vi "Open UI.vi"(11 "Open UI in":refnum<class "Open UI.lvclass">) -> (0 "error out":errorcluster, 3 "Open UI out":refnum<class "Open UI.lvclass">)   [LabVIEW 2021, in "Open UI.lvlib" / "Open UI.lvclass"]
uses:
  Open UI.lvclass
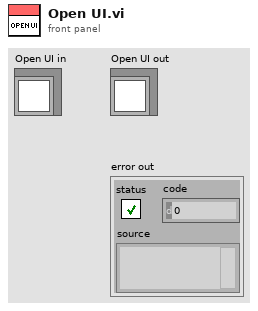
[diagram p1: front panel]
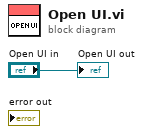
[diagram p0: block diagram]
diagram:
  "Open UI out" <- "Open UI in"
